vi "Format Instrument Identifier.vi"(10 "Identifier":string) -> (2 "Formatted Identifier":string)   [LabVIEW 2025, in "Instrument Manager AE.lvlib"]
uses:
  Instrument Manager AE.lvlib
  <vilib>/Utility/error.llb/Trim Whitespace One-Sided.vi
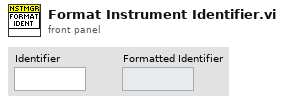
[diagram p1: front panel]
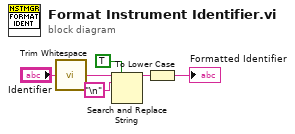
[diagram p0: block diagram]
diagram:
  n1 = call <vilib>:"Trim Whitespace.vi"("string"="Identifier") -> ("trimmed string"=w1:string)  [unwired: 1 in]
  n2 = Search and Replace String(replace all?=TRUE ("replace all? (F)"), input string=w1, search string="\n") -> (result string=w4:string)  [unwired: 5 in, 3 out]
  n3 = To Lower Case(string=w4) -> (all lower case string=→"Formatted Identifier":string)
